vi "AI to Newtons.vi"(1 "Sensor Reference":T1, 2 "AI 0-5":dbl[](array[numeric])=[0.0, 0.0, 0.0, 0.0, 0.0, 0.0]) -> (0 "Force (N)":dbl format="%.2f")   [LabVIEW 2011]
uses:
  ATI Force Sensor.ctl
  <vilib>/Analysis/baseanly.llb/Real Dot Product.vi
  <vilib>/Analysis/NI_AALBase.lvlib
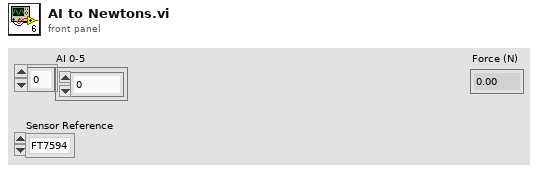
[diagram p1: front panel]
types:
  T1 = typedef "ATI Force Sensor.ctl" = enum16{"FT7594", "FT10263"}
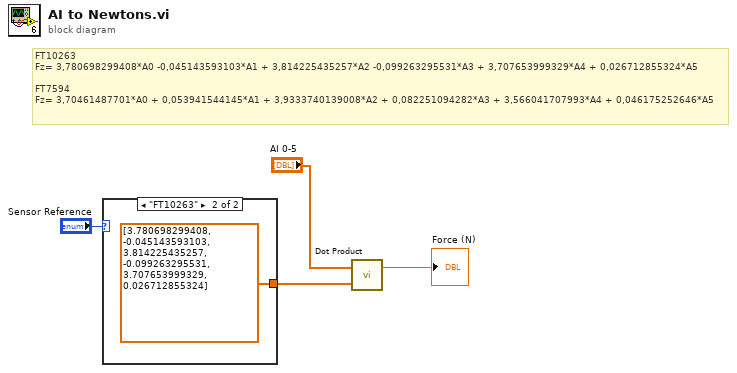
[diagram p0: block diagram]
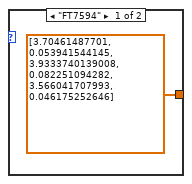
[diagram p2: hidden frame]
diagram:
  # "FT10263\nFz= 3,780698299408*A0 -0,045143593103*A1 + 3,814225435257*A2 -0,099263295531*A3 + 3,707653999329*A4 + 0,026712855324*A5\n\nFT7594\nFz= 3,70461487701*A0 + 0,053941544145*A1 + 3,9333740139008*A2 + 0,082251094282*A3 + 3,566041707993*A4 + 0,046175252646*A5"
  n1 = case shown="\"FT10263\"" "Sensor Reference" {
    tunnel: [dbl[] [3.70461487701, 0.053941544145, 3.9333740139008, 0.082251094282, 3.566041707993, 0.046175252646] ("AI 0-5") dbl[] [3.780698299408, -0.045143593103, 3.814225435257, -0.099263295531, 3.707653999329, 0.026712855324] ("AI 0-5")] -> w3
    frame "FT7594" {
    }
    frame "FT10263" {
    }
  }
  n2 = call-poly <vilib>:"Dot Product.vi"("Y Vector"=w3, "X Vector"="AI 0-5") -> ("X * Y"=→"Force (N)":dbl)  [unwired: 1 out]
